vi "KE6221 -- Get Wave Trig Link In Line.vi"(0 "Resource In":refnum<visa-resource-name>, 1 "Check For SCPI Errors? (T)":bool=TRUE, 11 "error in (no error)":errorcluster) -> (4 "Resource Out (dupl)":refnum<visa-resource-name>, 8 "Trig Link In Line":T1=enum."1", 15 "error out":errorcluster)   [LabVIEW 2019, in "Keithley 622x.lvlib"]
uses:
  Keithley 622x.lvlib
  Typedefs/KE6221 -- Wave Extern Trig Link In Line.ctl
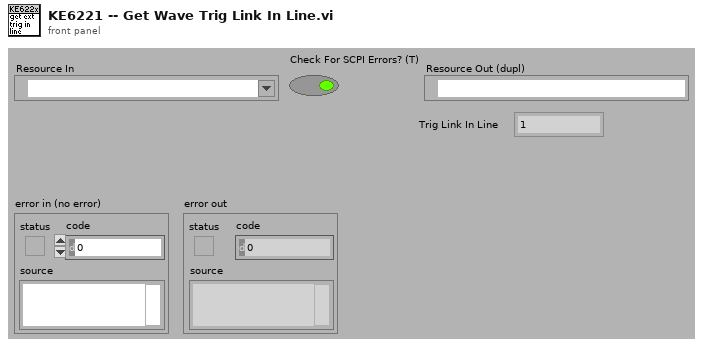
[diagram p1: front panel]
types:
  T1 = typedef "Keithley 622x.lvlib/KE6221 -- Wave Extern Trig Link In Line.ctl" = enum16{"None", "1", "2", "3", "4", "5", "6"}
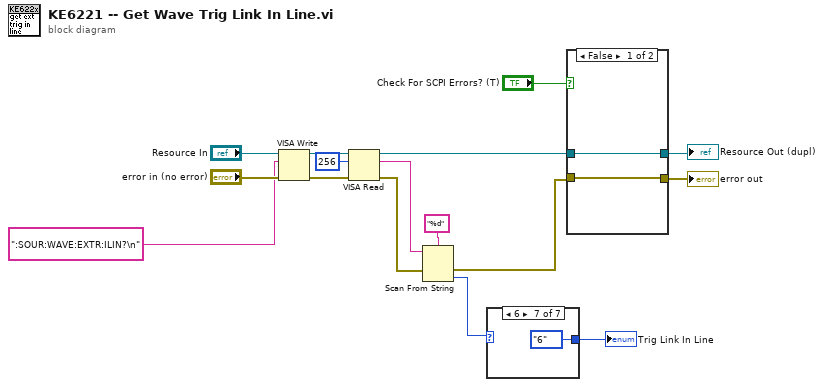
[diagram p0: block diagram]
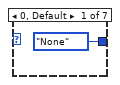
[diagram p2: hidden frame]
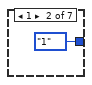
[diagram p3: hidden frame]
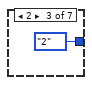
[diagram p4: hidden frame]
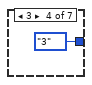
[diagram p5: hidden frame]
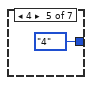
[diagram p6: hidden frame]
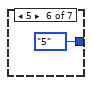
[diagram p7: hidden frame]
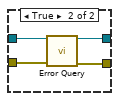
[diagram p8: hidden frame]
diagram:
  n1 = VISA Write(VISA resource name="Resource In", write buffer=":SOUR:WAVE:EXTR:ILIN?\n" ("format string"), error in (no error)="error in (no error)") -> (VISA resource name out=w10:refnum<visa-resource-name>, error out=w9:errorcluster)  [unwired: 1 out]
  n2 = VISA Read(VISA resource name=w10, byte count=u32 256, error in (no error)=w9) -> (VISA resource name out=w3:refnum<visa-resource-name>, read buffer=w5:string, error out=w7:errorcluster)  [unwired: 1 out]
  n3 = Scan From String(format string="%d", input string=w5, error in=w7) -> (error out=w4:errorcluster, output 1=w2:i32)  [unwired: 2 in, 2 out]
  n4 = case shown="6" w2 {
    tunnel: [KE6221_--_Wave_Extern_Trig_Link_In_Line."None" ("Trig In Line") KE6221_--_Wave_Extern_Trig_Link_In_Line."1" ("Trig In Line") KE6221_--_Wave_Extern_Trig_Link_In_Line."2" ("Trig In Line") KE6221_--_Wave_Extern_Trig_Link_In_Line."3" ("Trig In Line") KE6221_--_Wave_Extern_Trig_Link_In_Line."4" ("Trig In Line") KE6221_--_Wave_Extern_Trig_Link_In_Line."5" ("Trig In Line") KE6221_--_Wave_Extern_Trig_Link_In_Line."6" ("Trig In Line")] -> w1
    frame 0, Default {
    }
    frame 1 {
    }
    frame 2 {
    }
    frame 3 {
    }
    frame 4 {
    }
    frame 5 {
    }
    frame 6 {
    }
  }
  "Trig Link In Line" <- w1
  n5 = case shown="False" "Check For SCPI Errors? (T)" {
    tunnel: w3 -> [w25 w29]
    tunnel: w4 -> [w24 w28]
    tunnel: [w24 w27] -> w12
    tunnel: [w25 w26] -> w13
    frame False {
    }
    frame True {
      n6 = call "Error Query.vi"("VISA Resource In"=w29, "error in (no error)"=w28) -> ("VISA Resource Out (dupl)"=w26:refnum<visa-resource-name>, "error out"=w27:errorcluster)  [unwired: 10 in, 2 out]
    }
  }
  "Resource Out (dupl)" <- w13
  "error out" <- w12
